vi "reverseEndian32bit.vi"(8 "error in":errorcluster, 11 "In":string) -> (0 "error out":errorcluster, 3 "Out":string)   [LabVIEW 2018]
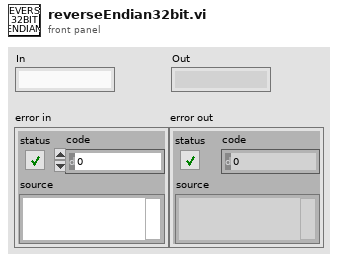
[diagram p1: front panel]
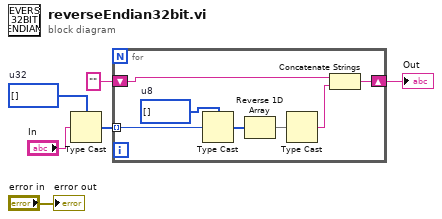
[diagram p0: block diagram]
diagram:
  w3 = u32[] []  # u32
  n1 = Type Cast(type=w3, x="In") -> (*(type *) &x=w4:u32[])
  n2 = for {
    tunnel: w4 -> [w13] mode=indexing
    shift-right: [w8] -> w6
    shift-left: "" -> [w7]
    w12 = u8[] []  # u8
    n3 = Type Cast(type=w12, x=w13) -> (*(type *) &x=w11:u8[])
    n4 = Reverse 1D Array(array=w11) -> (reversed array=w10:u8[])
    n5 = Type Cast(x=w10) -> (*(type *) &x=w9:string)  [unwired: 1 in]
    n6 = Concatenate Strings(w7, w9) -> (w8:string)
  }
  "Out" <- w6
  "error out" <- "error in"
